vi "Rinocloud_pagination.vi"(3 "error in (no error)":errorcluster, 5 "HTTP body":string) -> (0 "error out":errorcluster, 2 "pagination parameters":T1)   [LabVIEW 2011]
uses:
  i3 JSON/i3-json.lvlib
  i3 JSON/JSON Parsing/Get Object Parameter Files/Get Object Parameter - Numeric.vi
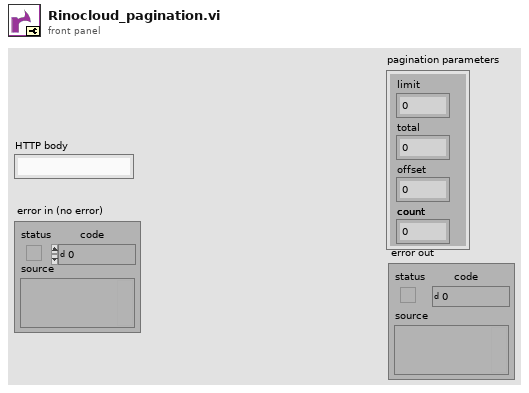
[diagram p1: front panel]
types:
  T1 = cluster{"limit":dbl, "total":dbl, "offset":dbl, "count":dbl}
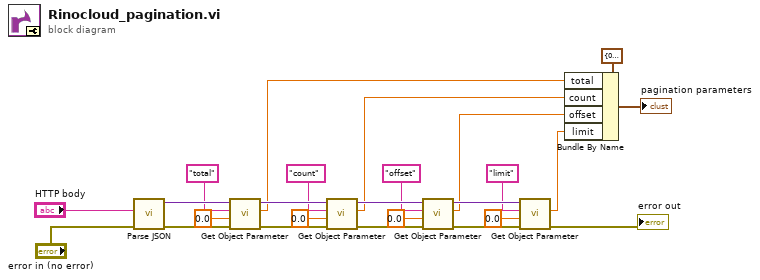
[diagram p0: block diagram]
diagram:
  n1 = call "Parse JSON.vi"("error in (no error)"="error in (no error)", "JSON String"="HTTP body") -> ("error out"=w17:errorcluster, "JSON Tree"=w23:variant)  [unwired: 6 in, 2 out]
  n2 = call-poly "Get Object Parameter.vi"("error in (no error)"=w17, "Default Value if JSON Null"=0.0, "Parameter Name"="total", "JSON Tree In (JSON Object)"=w23) -> ("error out"=w16:errorcluster, "Double Value"=w4:dbl, "JSON Tree Out Passthrough"=w22:variant)  [unwired: 4 in, 1 out]
  n3 = call-poly "Get Object Parameter.vi"("error in (no error)"=w16, "Default Value if JSON Null"=0.0, "Parameter Name"="count", "JSON Tree In (JSON Object)"=w22) -> ("error out"=w15:errorcluster, "Double Value"=w3:dbl, "JSON Tree Out Passthrough"=w21:variant)  [unwired: 4 in, 1 out]
  n4 = call-poly "Get Object Parameter.vi"("error in (no error)"=w15, "Default Value if JSON Null"=0.0, "Parameter Name"="offset", "JSON Tree In (JSON Object)"=w21) -> ("error out"=w14:errorcluster, "Double Value"=w2:dbl, "JSON Tree Out Passthrough"=w20:variant)  [unwired: 4 in, 1 out]
  n5 = call-poly "Get Object Parameter.vi"("error in (no error)"=w14, "Default Value if JSON Null"=0.0, "Parameter Name"="limit", "JSON Tree In (JSON Object)"=w20) -> ("error out"=→"error out":errorcluster, "Double Value"=w1:dbl)  [unwired: 4 in, 2 out]
  n6 = Bundle By Name(cluster=T1 {"limit"=0.0, "total"=0.0, "offset"=0.0, "count"=0.0} ("pagination parameters 2"), "total"=w4, "count"=w3, "offset"=w2, "limit"=w1) -> (→"pagination parameters":T1)
